vi "CallWrite.vi"(6 "Time out?":u8, 8 "error in (no error)":errorcluster, 10 "Data":u8, 11 "FPGA VI引用输入":refnum<k20>) -> (0 "error out":errorcluster, 3 "FPGA VI引用输出":refnum<k20>)   [LabVIEW 2015]
uses:
  <vilib>/Utility/error.llb/Error Cluster From Error Code.vi
  <vilib>/rvi/errors/niLvFpgaAdjustHostInterfaceError.vi
  <vilib>/rvi/interface/nirviReadWriteControl/nirviReadWriteControl.xnode
  <vilib>/rvi/interface/Simulation/niFpgaSimulationCallBeginRW.vi
  NiFpgaLv.dll
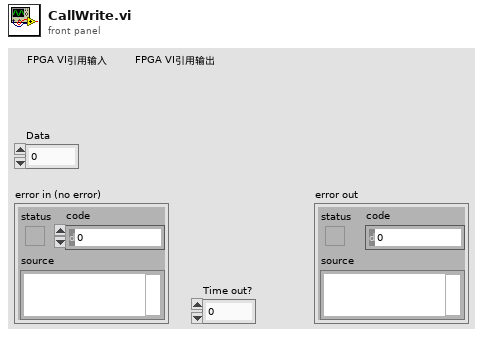
[diagram p1: front panel]
types:
  T1 = enum8{"IDLE", "SetIDLE", "Config", "Arm", "Read", "Write", "AutoRead"}
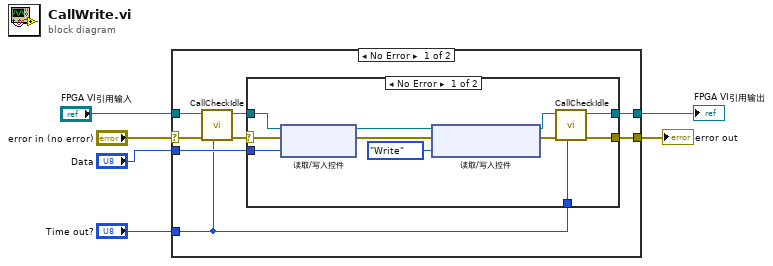
[diagram p0: block diagram]
diagram:
  n1 = case shown="No Error" "error in (no error)" {
    selector: "error in (no error)" -> [w12 w29]
    tunnel: [w13 w29] -> w6
    tunnel: "Data" -> [w14 _]
    tunnel: "Time out?" -> [w10 _]
    tunnel: "FPGA VI引用输入" -> [w8 w28]
    tunnel: [w7 w28] -> w1
    frame No Error {
      n2 = call "CallCheckIdle.vi"("Time out?"=w10, "error in (no error)"=w12, "FPGA VI引用输入"=w8) -> ("error out"=w11:errorcluster, "FPGA VI引用输出"=w9:refnum<k20>)  [unwired: 7 in]
      n3 = case shown="No Error" w11 {
        selector: w11 -> [w22 w27]
        tunnel: w14 -> [w23 _]
        tunnel: [w21 w27] -> w13
        tunnel: w10 -> [w19 _]
        tunnel: w9 -> [w16 w26]
        tunnel: [w15 w26] -> w7
        frame No Error {
          n4 = xnode "读取/写入控件"("FPGA VI Reference In"=w16, "error in"=w22, "WriteData"=w23) -> ("FPGA VI Reference Out"=w24:refnum<k20>, "error out"=w25:errorcluster)
          n5 = xnode "读取/写入控件"("FPGA VI Reference In"=w24, "error in"=w25, "ProtocolControl"=T1."Write") -> ("FPGA VI Reference Out"=w17:refnum<k20>, "error out"=w20:errorcluster)
          n6 = call "CallCheckIdle.vi"("Time out?"=w19, "error in (no error)"=w20, "FPGA VI引用输入"=w17) -> ("error out"=w21:errorcluster, "FPGA VI引用输出"=w15:refnum<k20>)  [unwired: 7 in]
        }
        frame Error {
        }
      }
    }
    frame Error {
    }
  }
  "error out" <- w6
  "FPGA VI引用输出" <- w1
